vi "test_SessionReservationInfo_ReserveSessions_SessionReservedBooleanTrue.vi"(8 "error in":errorcluster) -> (0 "error out":errorcluster, 2 "result":string, 3 "pass":bool)   [LabVIEW 2021, in "MeasurementServerTests.lvlib" / "Session Reservation Tests.lvlib"]
uses:
  Session Reservation Tests.lvlib
  gRPC/Generated APIs/ni/measurementlink/sessionmanagement/v1/RPC Messages/ni_measurementlink_PinMapContext.ctl
  Runtime/Clients/Session Management V1/Session Reservation/Session Reservation.lvclass/Session Reservation.ctl
  Runtime/Clients/Session Management V1/Session Reservation/Merge Invalid DVR Error.vi
  Helpers/Pin Map XML Strings Global.vi
  Runtime/Clients/Session Management V1/Session Reservation/Is DVR Valid.vi
  Runtime/Measurements/Helpers/Error Strings Global Internal.vi
  <vilib>/Utility/error.llb/Error Cluster From Error Code.vi
  gRPC/Generated APIs/ni/measurementlink/sessionmanagement/v1/ni.measurementlink.sessionmanagement.v1.api.lvlib
  MeasurementServerTests.lvlib
  Runtime/Clients/Session Management V1/Session Reservation/Session Reservation.lvclass
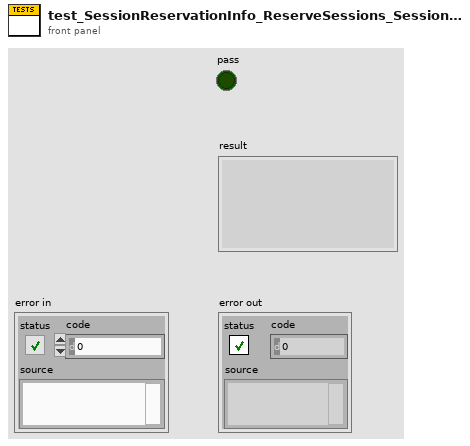
[diagram p1: front panel]
types:
  T1 = typedef "ni.measurementlink.sessionmanagement.v1.api.lvlib/ni_measurementlink_PinMapContext.ctl" = cluster{"pin_map_id":string, "sites":i32[]}
  T2 = typedef "ni.measurementlink.sessionmanagement.v1.api.lvlib/ni_measurementlink_sessionmanagement_v1_SessionInformation.ctl" = cluster{"session":T3, "resource_name":string, "channel_list":string, "instrument_type_id":string, "session_exists":bool, "session_reserved":bool, "channel_mappings":T4[], "annotations":T5[]}
  T3 = typedef "ni.measurementlink.sessionmanagement.v1.api.lvlib/nidevice_grpc_Session.ctl" = cluster{"name":string}
  T4 = typedef "ni.measurementlink.sessionmanagement.v1.api.lvlib/ni_measurementlink_sessionmanagement_v1_ChannelMapping.ctl" = cluster{"pin_or_relay_name":string, "site":i32, "channel":string, "multiplexer_resource_name":string, "multiplexer_route":string}
  T5 = typedef "ni.measurementlink.sessionmanagement.v1.api.lvlib/ni_measurementlink_sessionmanagement_v1_SessionInformation_AnnotationsEntry.ctl" = cluster{"key":string, "value":string}
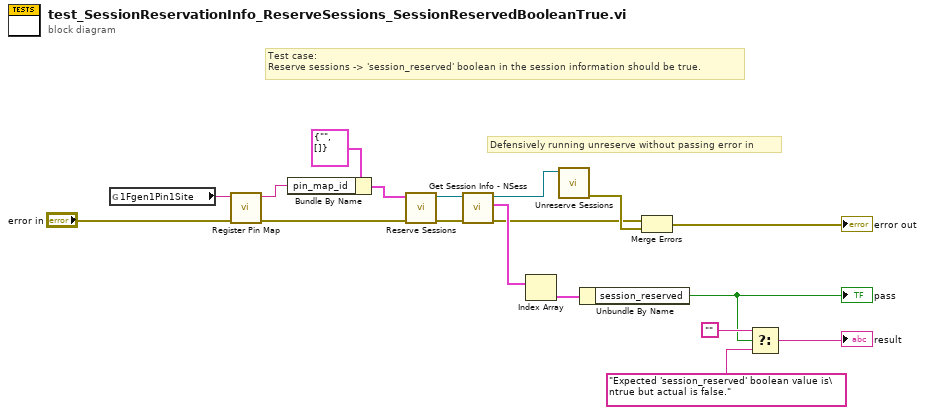
[diagram p0: block diagram]
diagram:
  # "Defensively running unreserve without passing error in"
  # "Test case:\nReserve sessions -> 'session_reserved' boolean in the session information should be true."
  n1 = global read "Pin Map XML Strings Global.vi" "1Fgen1Pin1Site"() -> (w7:string)
  n2 = call "Register Pin Map.vi"("error in"="error in", "pin map xml"=w7) -> ("error out"=w5:errorcluster, "pin map id"=w8:string)  [unwired: 8 in]
  n3 = Bundle By Name(cluster=T1 {"pin_map_id"="", "sites"=[]} ("pin map context"), "pin_map_id"=w8) -> (w17:T1)
  n4 = call "Reserve Sessions.vi"("error in"=w5, "pin map context"=w17) -> ("error out"=w16:errorcluster, "session reservation out"=w15:refnum<class "Session Reservation.lvclass">)  [unwired: 8 in]
  n5 = call "Get Session Info - NSess .vi"("error in"=w16, "session reservation in"=w15) -> ("error out"=w11:errorcluster, "sessions info"=w14:T2[], "session reservation out"=w13:refnum<class "Session Reservation.lvclass">)  [unwired: 7 in]
  n6 = Index Array(array=w14) -> (element=w9:T2)  [unwired: 1 in]
  n7 = call "Unreserve Sessions.vi"("session reservation in"=w13) -> ("error out"=w12:errorcluster)  [unwired: 10 in]
  n8 = Unbundle By Name(w9) -> ("session_reserved"=w1:bool)
  "pass" <- w1
  n9 = Merge Errors(w11, w12) -> (→"error out":errorcluster)
  n10 = Select(t="", s=w1, f="Expected 'session_reserved' boolean value is\ntrue but actual is false.") -> (s? t:f=→"result":string)
